vi "Example_DVR.vi"() -> ()   [LabVIEW 2020, in "OpenLvVision_Image.lvlib"]
uses:
  OpenLvVision_Image.lvlib
  Management/TypeDef/ImageType.ctl
  DataAccess/Dvr/ImageToDvrU32_2D.vi
  Management/Management.lvlib
  File/File.lvlib
  DataAccess/DataAccess.lvlib
panel:
  in  "Image Path":path
  in  "ChangeColor":bool
  in  "Color":u32(colorbox)
  out "Image":T1(plugin-control)
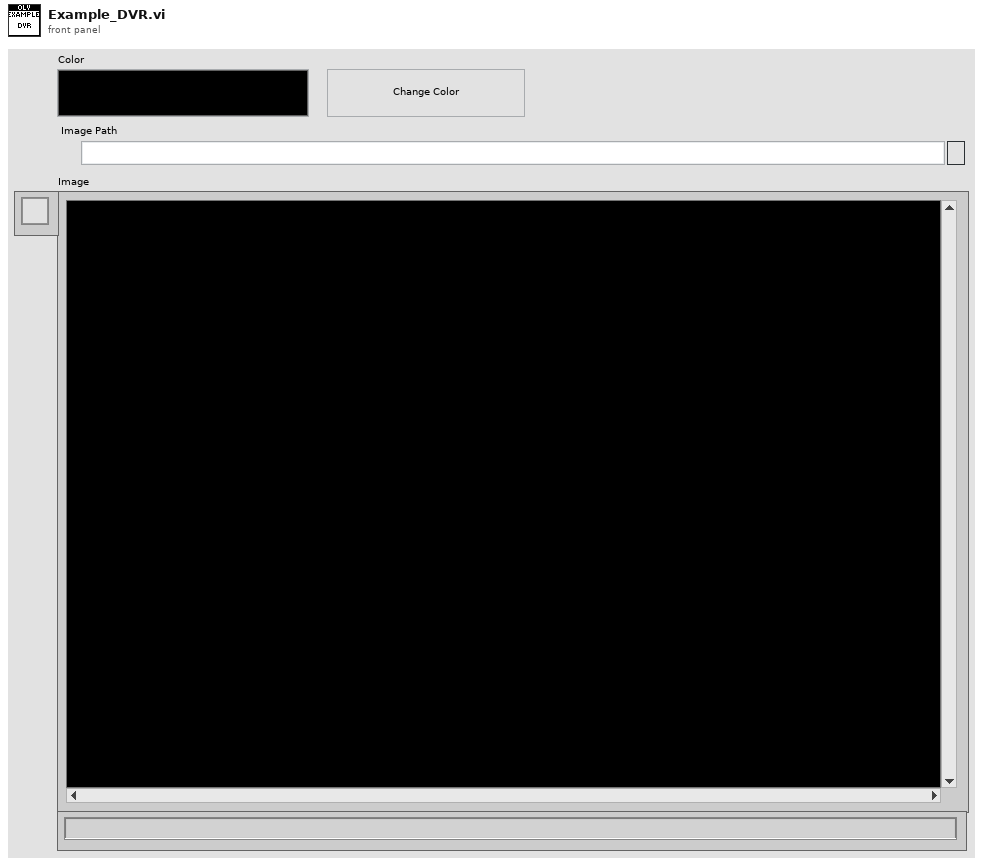
[diagram p1: front panel]
types:
  T1 = typedef "IMAQ Image.ctl" = refnum<image>
  T2 = typedef "OpenLvVision_Image.lvlib/Management.lvlib/ImageType.ctl" = enum16{"Mono U8", "Mono U16", "Mono I16", "Mono SGL", "Color U32", "Color U64", "Complex CSG"}
  T3 = typedef "OpenLvVision_Image.lvlib/Management.lvlib/Image.ctl" = refnum<image>
  T4 = cluster{"Global Rectangle":i32[], "Contours":cluster{"Contour Type":u32, "ROI Type":u32, "Points":i32[]}[]}
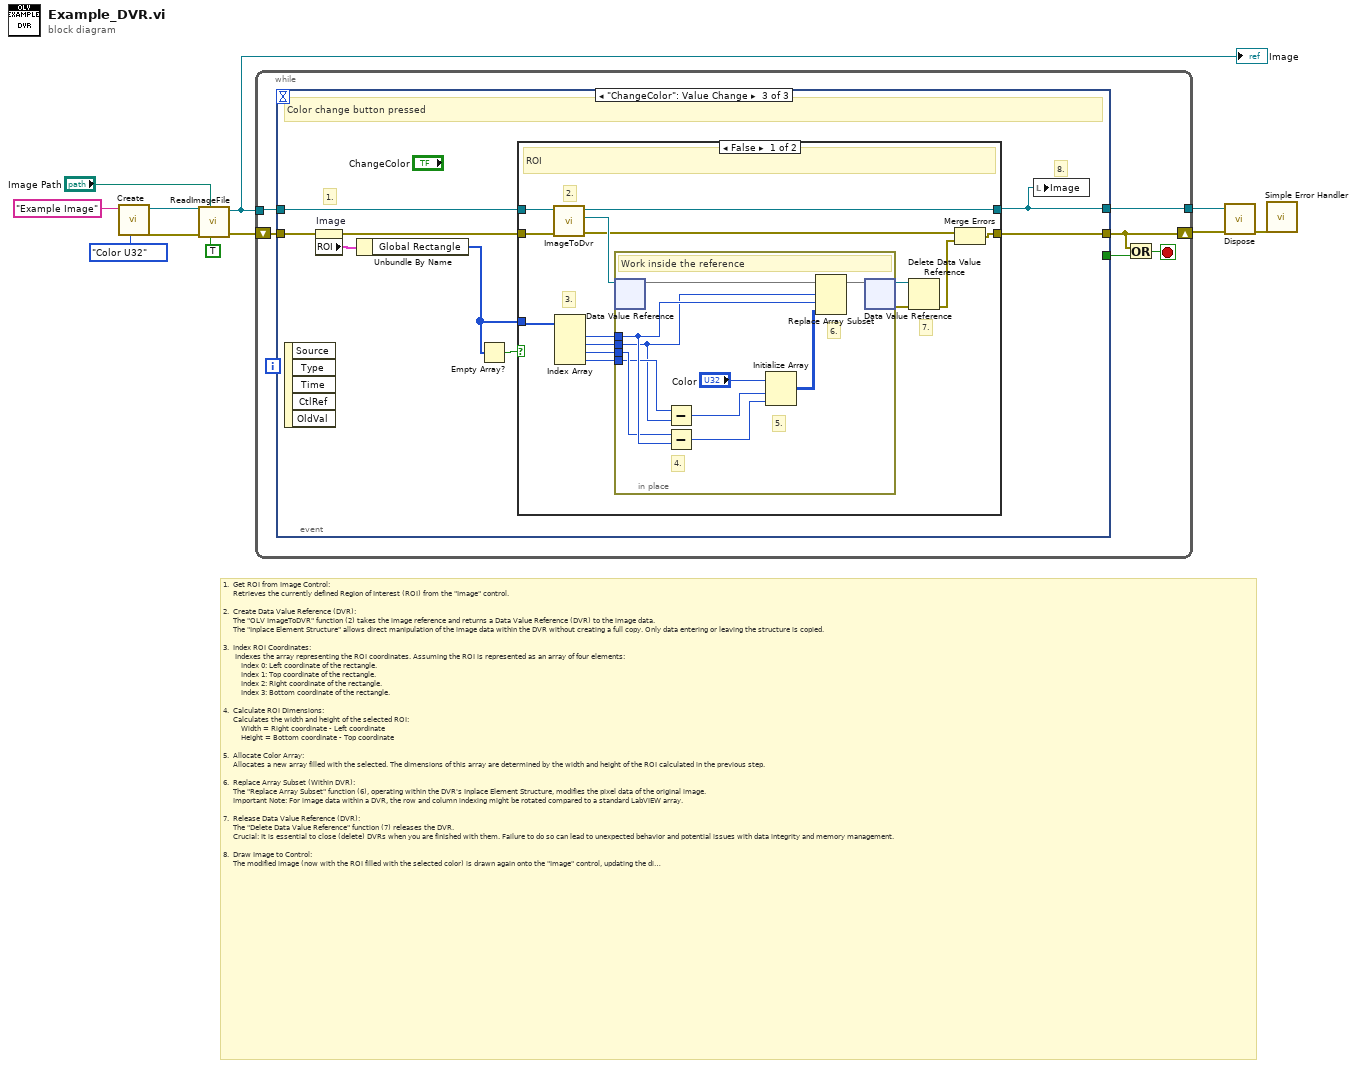
[diagram p0: block diagram]
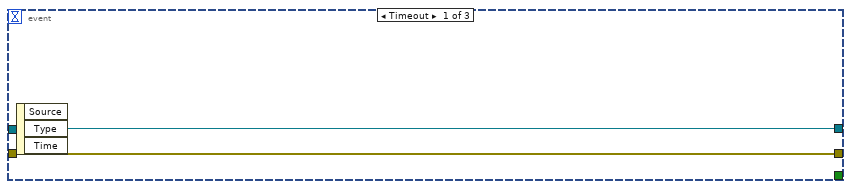
[diagram p2: hidden frame]
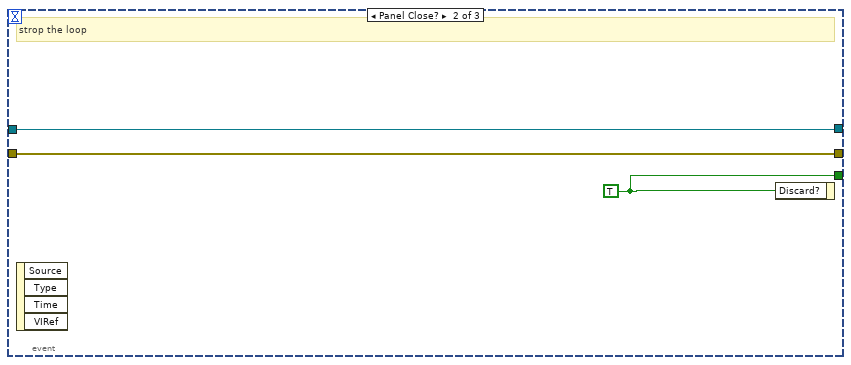
[diagram p3: hidden frame]
diagram:
  # "1.  Get ROI from Image Control:\n     Retrieves the currently defined Region of Interest (ROI) from the \"Image\" control.\n\n2.  Create Data Value Reference (DVR):\n     The \"OLV ImageToDVR\" function (2) takes the image reference and returns a Data Value Reference (DVR) to the image data.\n     The \"Inplace Element Structure\" allows direct manipulation of the image data within the DVR without creating a full copy. Only data entering or leaving the structure is copied.\n\n3.  Index ROI Coordinates:\n      Indexes the array representing the ROI coordinates. Assuming the ROI is represented as an array of four elements:\n         Index 0: Left coordinate of the rectangle.\n         Index 1: Top coordinate of the rectangle.\n         Index 2: Right coordinate of the rectangle.\n         Index 3: Bottom coordinate of the rectangle.\n\n4.  Calculate ROI Dimensions:\n     Calculates the width and height of the selected ROI:\n         Width = Right coordinate - Left coordinate\n         Height = Bottom coordinate - Top coordinate\n\n5.  Allocate Color Array:\n     Allocates a new array filled with the selected. The dimensions of this array are determined by the width and height of the ROI calculated in the previous step. \n\n6.  Replace Array Subset (Within DVR):\n     The \"Replace Array Subset\" function (6), operating within the DVR's Inplace Element Structure, modifies the pixel data of the original image.\n     Important Note: For image data within a DVR, the row and column indexing might be rotated compared to a standard LabVIEW array.\n\n7.  Release Data Value Reference (DVR):\n     The \"Delete Data Value Reference\" function (7) releases the DVR.\n     Crucial: It is essential to close (delete) DVRs when you are finished with them. Failure to do so can lead to unexpected behavior and potential issues with data integrity and memory management.\n\n8.  Draw Image to Control:\n     The modified image (now with the ROI filled with the selected color) is drawn again onto the \"Image\" control, updating the displayed image with the changes made within the DVR."
  n1 = call "Create.vi"("Image Type"=ImageType."Color U32", "Image Name"="Example Image") -> ("error out"=w8:errorcluster, "Image Reference Out"=w9:T3)  [unwired: 8 in]
  n2 = call "ReadImageFile.vi"("Use File Path Image Type"=TRUE, "File Path"="Image Path", "error in"=w8, "Image Reference In"=w9) -> ("error out"=w6:errorcluster, "Image Reference Out"=w5:T3)  [unwired: 3 in, 3 out]
  "Image" <- w5
  n3 = while {
    tunnel: w5 -> [w17]
    shift-right: [w14] -> w3
    shift-left: w6 -> [w16]
    tunnel: [w15] -> w4
    stop <- w13 stop-if-true
    n4 = event shown="[2] \"ChangeColor\": Value Change" {
      selector: _ -> [_ _ _]
      dyn-events: _ -> [_ _ _]
      timeout: _ -> [_ _ _]
      tunnel: w17 -> [w19 w22 w27]
      tunnel: w16 -> [w18 w21 w30]
      tunnel: [w18 w21 w24] -> w14
      tunnel: [w19 w22 w23] -> w15
      tunnel: [_ w20 _] -> w12
      event Timeout {
        n5 = event-data() -> ()  [unwired: 1 in, 3 out]
      }
      event Panel Close? {
        w20 = TRUE
        # "strop the loop"
        n6 = event-data() -> ()  [unwired: 1 in, 4 out]
        n7 = event-data("Discard?"=w20) -> ()  [unwired: 1 in, 1 out]
      }
      event "ChangeColor": Value Change {
        # "8."
        # "1."
        # "Color change button pressed"
        n8 = event-data() -> ()  [unwired: 1 in, 5 out]
        n9 = property on="Image" class="ImageControl"(error in=w30) -> (error out=w26:errorcluster, "ROI"=w29:T4)  [unwired: 1 in, 1 out]
        n10 = Unbundle By Name(w29) -> ("Global Rectangle"=w25:i32[])
        n11 = Empty Array?(array=w25) -> (empty?=w28:bool)
        n12 = case shown="False" w28 {
          tunnel: w27 -> [w44 w56]
          tunnel: w26 -> [w43 w55]
          tunnel: w25 -> [w41 _]
          tunnel: [w36 w56] -> w23
          tunnel: [w31 w55] -> w24
          frame False {
            # "7."
            # "3."
            # "2."
            # "ROI"
            n13 = call-poly "ImageToDvr.vi"("error in"=w43, "Image Reference In"=w44) -> ("error out"=w35:errorcluster, "EDVR 2D U32"=w42:refnum<data-value>, "Image Reference Out"=w36:T3)  [unwired: 6 in, 1 out]
            n14 = Index Array(array=w41) -> (element #1=w40:i32, element #2=w39:i32, element #3=w38:i32, element #4=w37:i32)  [unwired: 4 in]
            n15 = in-place {
              in-place-border: w40 -> [w51]
              in-place-border: w39 -> [w45]
              in-place-border: w38 -> [w50]
              in-place-border: w37 -> [w46]
              # "6."
              # "5."
              # "4."
              # "Work inside the reference"
              n16 = in-place-dvr #1(w42) -> (w54:u32[][])  [unwired: 1 out]
              n17 = Subtract(x=w46, y=w45) -> (x-y=w49:i32)
              n18 = Subtract(x=w50, y=w51) -> (x-y=w48:i32)
              n19 = Initialize Array("Color", w49, w48) -> (w52:u32[][])
              n20 = Replace Array Subset(array=w54, new element=w52, index (row)=w45, index (col)=w51) -> (w53:u32[][])
              n21 = in-place-dvr #1(w53) -> (w33:refnum<data-value>, w34:errorcluster)
            }
            n22 = Delete Data Value Reference(data value reference=w33, error in=w34) -> (error out=w32:errorcluster)  [unwired: 1 out]
            n23 = Merge Errors(w35, w32) -> (w31:errorcluster)
          }
          frame True {
            # "Roi empty"
          }
        }
        n24 = local write "Image"(w23) -> ()
      }
    }
    n25 = Or(x=w14, y=w12) -> (x .or. y?=w13:bool)
  }
  n26 = call "Dispose.vi"("error in"=w3, "Image Reference In"=w4) -> ("error out"=w2:errorcluster)  [unwired: 9 in]
  n27 = call <vilib>:"Simple Error Handler.vi"("error in (no error)"=w2) -> ()  [unwired: 4 in, 5 out]
